vi "SCT Launch Help.vi"(6 "feature pack info":T1, 8 "error in (no error)":errorcluster, 9 "Feature":i32, 10 "Variable Type":i32) -> (0 "error out":errorcluster)   [LabVIEW 2016]
uses:
  <resource>/dialog/variable/SCT Feature Pack Info.ctl
  <resource>/dialog/variable/SCT Message User Event.ctl
  <resource>/dialog/variable/SCT Message.ctl
  <vilib>/variable/Type Descriptor.ctl
  <resource>/dialog/variable/SCT Attributes.ctl
  <resource>/dialog/variable/SCT Attributes Event.ctl
  <vilib>/variable/NI_Variable.lvlib
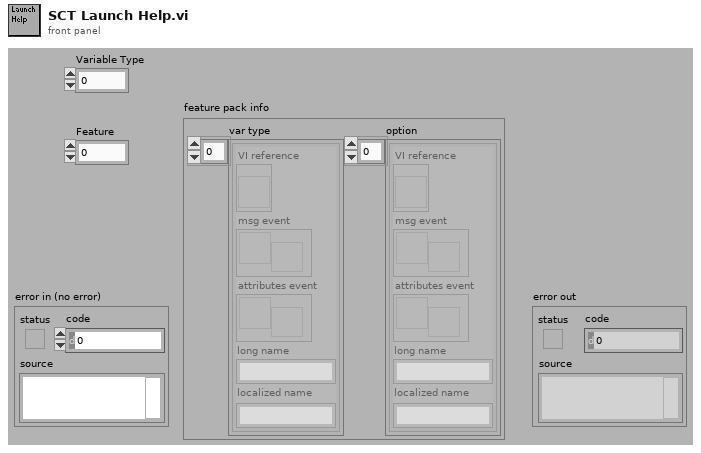
[diagram p1: front panel]
types:
  T1 = typedef "SCT Feature Pack Info.ctl" = cluster{"var type":cluster{"VI reference":refnum<vi>, "msg event":T2, "attributes event":T3, "long name":string, "localized name":string}[], "option":cluster{"VI reference":refnum<vi>, "msg event":T2, "attributes event":T3, "long name":string, "localized name":string}[]}
  T2 = typedef "SCT Message User Event.ctl" = refnum<user-event>
  T3 = typedef "SCT Attributes Event.ctl" = refnum<user-event>
  T4 = cluster{"VI reference":refnum<vi>, "msg event":T2, "attributes event":T3, "long name":string, "localized name":string}[]
  T5 = cluster{"VI reference":refnum<vi>, "msg event":T2, "attributes event":T3, "long name":string, "localized name":string}
  T6 = typedef "SCT Message.ctl" = cluster{"request type":enum16{"No Message", "New Data Type", "New Variable", "Request Values", "Shutdown", "Broadcast", "Show Help"}, "name":string, "type descriptor":T7, "scope":string, "attributes":T8, "broadcast value":variant}
  T7 = typedef "NI_Variable.lvlib/Type Descriptor.ctl" = cluster{"Variant":variant}
  T8 = typedef "SCT Attributes.ctl" = cluster{"name":string, "value":string, "ambiguous?":bool}[]
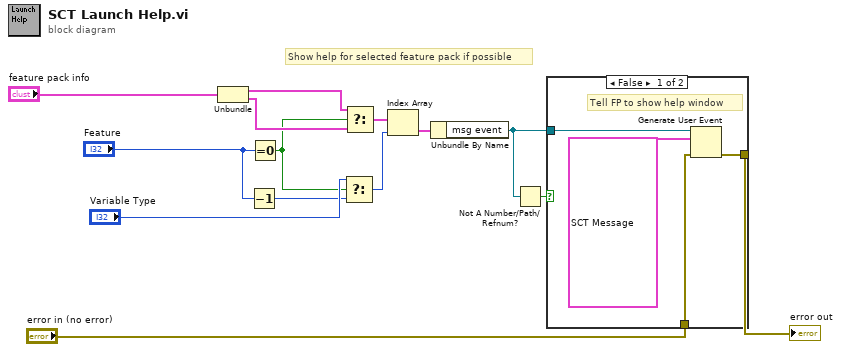
[diagram p0: block diagram]
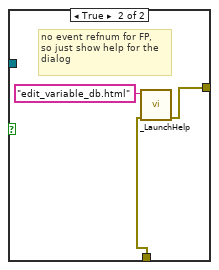
[diagram p2: hidden frame]
diagram:
  # "Show help for selected feature pack if possible"
  n1 = Unbundle("feature pack info") -> ("var type"=w8:T4, "option"=w7:T4)
  n2 = Decrement(x="Feature") -> (x-1=w5:i32)
  n3 = Equal To 0?(x="Feature") -> (x = 0?=w6:bool)
  n4 = Select(t="Variable Type", s=w6, f=w5) -> (s? t:f=w4:i32)
  n5 = Select(t=w8, s=w6, f=w7) -> (s? t:f=w3:T4)
  n6 = Index Array(array=w3, index=w4) -> (element=w9:T5)
  n7 = Unbundle By Name(w9) -> ("msg event"=w2:T2)
  n8 = Not A Number/Path/Refnum?(number/path/refnum=w2) -> (NaN/Path/Refnum?=w1:bool)
  n9 = case shown="False" w1 {
    tunnel: w2 -> [w18 _]
    tunnel: "error in (no error)" -> [w16 w20]
    tunnel: [w15 w19] -> w10
    frame False {
      # "Tell FP to show help window"
      n10 = Generate User Event(user event=w18, event data cluster=T6 {"request type"=enum."Show Help", "name"="", "type descriptor"={"Variant"=variant}, "scope"="", "attributes"=[], "broadcast value"=variant} ("event data"), error in=w16) -> (error out=w15:errorcluster)  [unwired: 1 in, 1 out]
    }
    frame True {
      # "no event refnum for FP,\nso just show help for the\ndialog"
      n11 = call <helpdir>:"_LaunchHelp.vi"("error in (no error)"=w20, "HTML filename"="edit_variable_db.html") -> ("error out"=w19:errorcluster)  [unwired: 5 in]
    }
  }
  "error out" <- w10
